vi "Activate.vi"(8 "error in (no error)":errorcluster, 11 "Object License in":refnum<class "Software License Manager.lvclass">) -> (0 "error out":errorcluster, 1 "ok?":bool, 3 "Object License out":refnum<class "Software License Manager.lvclass">)   [LabVIEW 2025, in "SW License Manager.lvlib" / "Software License Manager.lvclass"]
uses:
  Software License Manager.lvclass
  Software License Manager.lvclass/Software License Manager.ctl
  Board/Board.lvclass/Board.ctl
  Properties/Read Website.vi
  Properties/Read Secret Key for License Verification Requests.vi
  Properties/Read Board.vi
  Board/Read Product ID.vi
  Board/Read Host Name.vi
  <vilib>/httpClient/POSTBuffer.vi
  Board/Board.lvclass
  <vilib>/httpClient/LabVIEWHTTPClient.lvlib
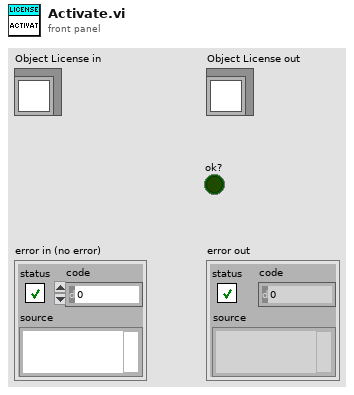
[diagram p1: front panel]
types:
  T1 = typedef "LabVIEWHTTPClient.lvlib/ClientHandle.ctl" = refnum<k1>
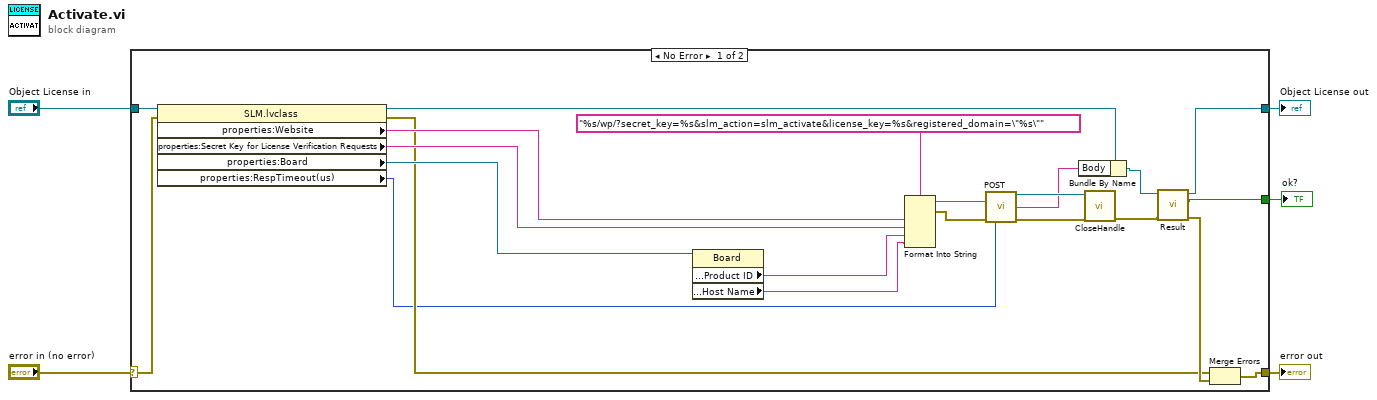
[diagram p0: block diagram]
diagram:
  n1 = case shown="No Error" "error in (no error)" {
    selector: "error in (no error)" -> [w8 w29]
    tunnel: [w21 w29] -> w4
    tunnel: [w13 w28] -> w2
    tunnel: "Object License in" -> [w20 w28]
    tunnel: [w14 _] -> w1
    frame No Error {
      n2 = property class="SLM.lvclass"(reference=w20, error in=w8) -> (reference out=w12:refnum<class "Software License Manager.lvclass">, error out=w7:errorcluster, "properties:Website"=w11:string, "properties:Secret Key for License Verification Requests"=w10:string, "properties:Board"=w9:refnum<class "Board.lvclass">, "properties:RespTimeout(us)"=w6:i32)
      n3 = property class="Board"(reference=w9) -> ("properties:Product ID"=w26:string, "properties:Host Name"=w25:string)  [unwired: 1 in, 2 out]
      n4 = Format Into String(format string="%s/wp/?secret_key=%s&slm_action=slm_activate&license_key=%s&registered_domain=\"%s\"", w11, w10, w26, w25) -> (resulting string=w18:string, error out=w22:errorcluster)  [unwired: 2 in]
      n5 = call-poly <vilib>:"POST.vi"("url"=w18, "error in (no error)"=w22, "timeout (10000)"=w6) -> ("client handle out"=w24:T1, "body"=w19:string, "error out"=w23:errorcluster)  [unwired: 9 in, 1 out]
      n6 = Bundle By Name(cluster=w12, "Body"=w19) -> (w17:refnum<class "Software License Manager.lvclass">)
      n7 = call <vilib>:"CloseHandle.vi"("client handle"=w24, "error in (no error)"=w23) -> ("error out"=w16:errorcluster)  [unwired: 13 in]
      n8 = call-dynamic "Result.vi"("error in (no error)"=w16, "Software License Manager in"=w17) -> ("error out"=w15:errorcluster, "ok?"=w14:bool, "Software License Manager out"=w13:refnum<class "Software License Manager.lvclass">)  [unwired: 6 in, 1 out]
      n9 = Merge Errors(w7, w15) -> (w21:errorcluster)
    }
    frame Error {
    }
  }
  "error out" <- w4
  "Object License out" <- w2
  "ok?" <- w1
